vi "DrawACard.vi"(10 "Player":T1, 11 "Game":T2) -> (2 "NewPlayer":T1, 3 "NewGame":T2)   [LabVIEW 2025]
uses:
  Controls/Player.ctl
  Controls/Game.ctl
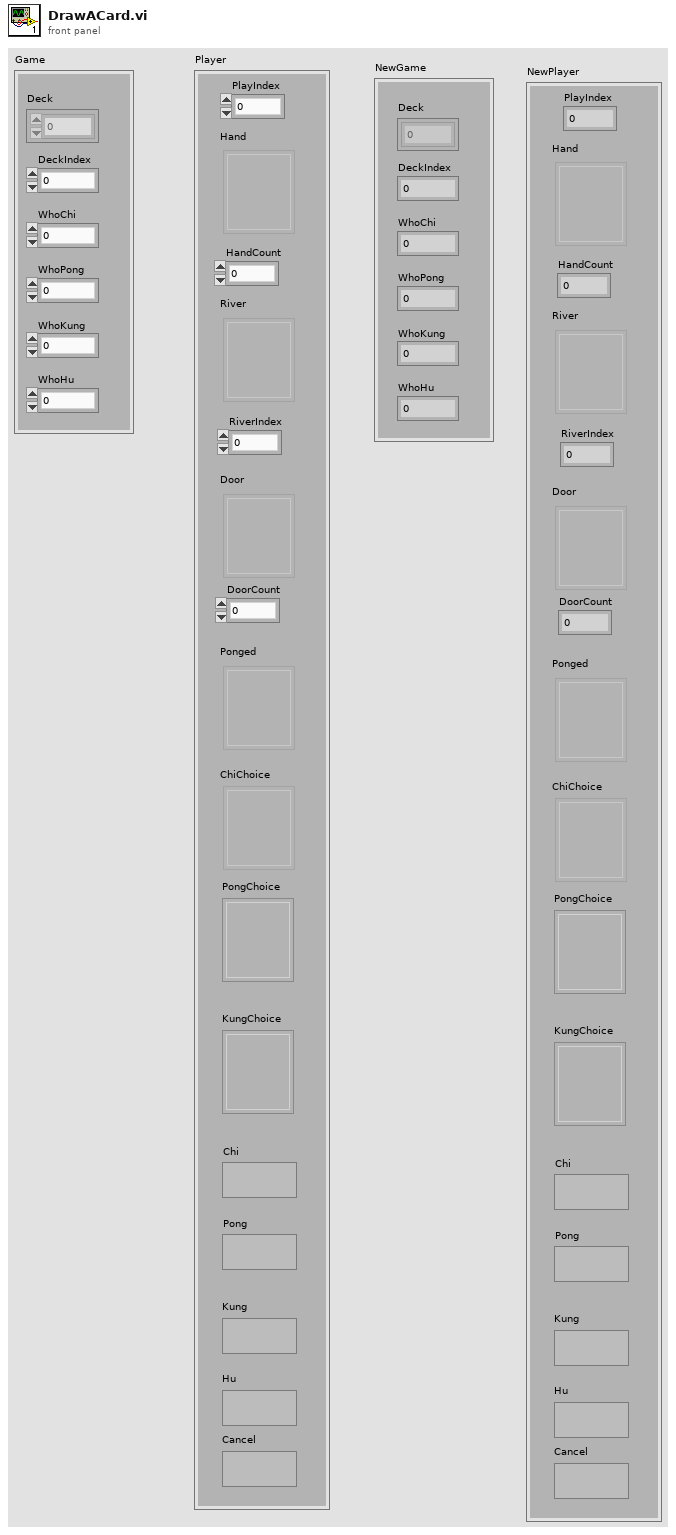
[diagram p1: front panel]
types:
  T1 = typedef "Player.ctl" = cluster{"PlayIndex":u16, "Hand":u16[], "HandCount":u16, "RiverIndex":u16, "Door":u16[], "DoorCount":u16, "Ponged":u16[], "ChiChoice":u16[][], "River":u16[][], "Chi":bool, "Pong":bool, "Kung":bool, "Hu":bool, "Cancel":bool, "PongChoice":u16, "KungChoice":u16}
  T2 = typedef "Game.ctl" = cluster{"DeckIndex":u16, "Deck":u16[], "WhoChi":u16, "WhoPong":u16, "WhoKung":u16, "WhoHu":u16}
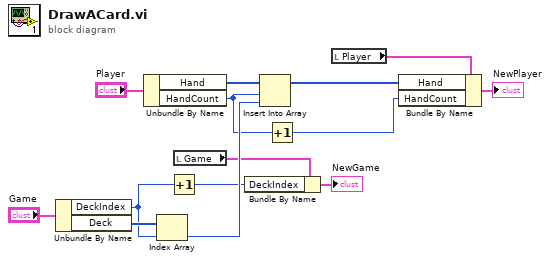
[diagram p0: block diagram]
diagram:
  n1 = Unbundle By Name("Game") -> ("DeckIndex"=w3:u16, "Deck"=w13:u16[])
  n2 = Unbundle By Name("Player") -> ("Hand"=w11:u16[], "HandCount"=w7:u16)
  n3 = Index Array(array=w13, index=w3) -> (element=w10:u16)
  n4 = Increment(x=w3) -> (x+1=w2:u16)
  n5 = local read "Game"() -> (w4:T2)
  n6 = Bundle By Name(cluster=w4, "DeckIndex"=w2) -> (→"NewGame":T2)
  n7 = Insert Into Array(array=w11, index=w7, new element=w10) -> (w1:u16[])
  n8 = Increment(x=w7) -> (x+1=w6:u16)
  n9 = local read "Player"() -> (w8:T1)
  n10 = Bundle By Name(cluster=w8, "Hand"=w1, "HandCount"=w6) -> (→"NewPlayer":T1)
